vi "to string.vi"(8 "error in":errorcluster, 11 "Thermo Channel configuration":refnum<class "Thermo Channel configuration.lvclass">) -> (0 "error out":errorcluster, 1 "data":string, 2 "version":string, 3 "Thermo Channel configuration out":refnum<class "Thermo Channel configuration.lvclass">)   [LabVIEW 2025, in "Thermo.lvlib" / "Thermo Channel configuration.lvclass"]
doc: "Provides an interface for saving a module configuration to a file or other serialized data source. It is recommended that all children of this class store data in two sets--data required for its own initialization, and any data required for parent initialization--and that each implementation uses the <b>Call Parent Method</b> primitive to serialize parent information.Copyright 2017 National Instruments Corporation\n\nLicensed under the Apache License, Version 2.0 (the \"License\"); you may not use this file except in compliance with the License. You may obtain a copy of the License at http://www.apache.org/licenses/LICENSE-2.0\nUnless required by applicable law or agreed to in writing, software distributed under the License is distributed on an \"AS IS\" BASIS, WITHOUT WARRANTIES OR CONDITIONS OF ANY KIND, either express or implied. See the License for the specific language governing permissions and limitations under the License."
uses:
  Thermo Channel configuration.lvclass
  C:/Users/Public/Documents/Sandia National Labs/TSS Plugin/Abstract Engine.lvlibp/Plugin/Abstract/Channel configuration/Channel configuration.lvclass
  Thermo Channel configuration.lvclass/Thermo Channel configuration.ctl
  Read Thermo Channel.vi
  Users/Public/Documents/Sandia National Labs/TSS Plugin/Abstract Engine.lvlibp/Plugin/Abstract/Channel configuration/Read Channel Setting.vi
  Users/Public/Documents/Sandia National Labs/TSS Plugin/Abstract Engine.lvlibp/Plugin/Abstract/Channel configuration/Channel configuration.lvclass
  Users/Public/Documents/Sandia National Labs/TSS Plugin/CEF.lvlibp/serializable configuration/CEF_serializable configuration.lvclass
  Users/Public/Documents/Sandia National Labs/TSS Plugin/CEF.lvlibp
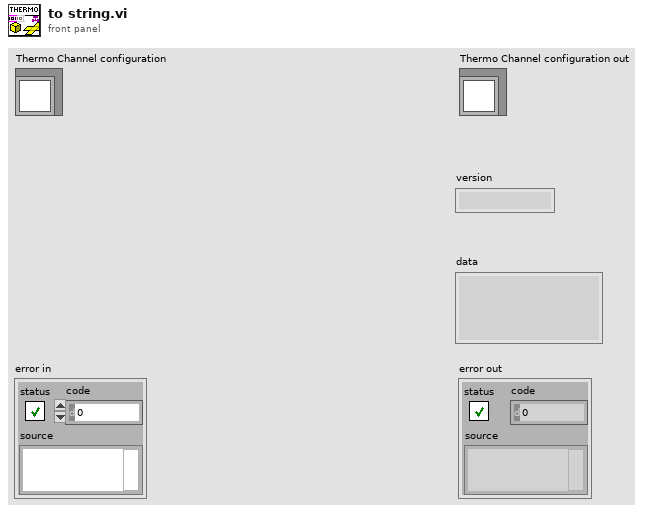
[diagram p1: front panel]
types:
  T1 = typedef "Thermo.lvlib/Thermo Channel configuration.lvclass/Channel Setting.ctl" = cluster{"Numeric":dbl, "Combo":string, "String":string, "Boolean":bool}
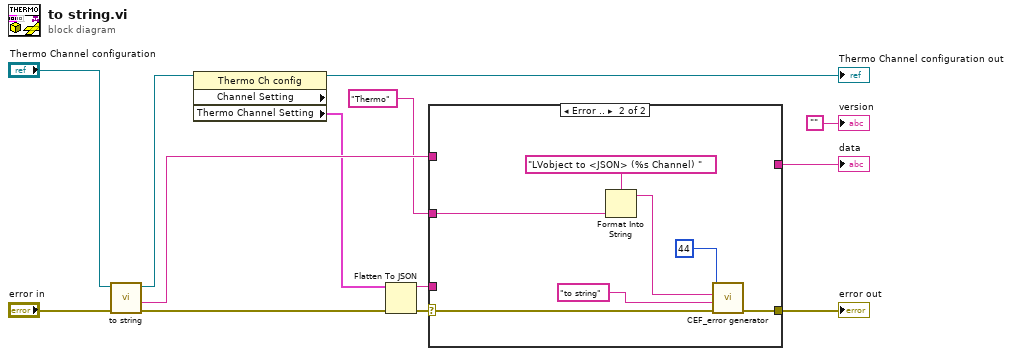
[diagram p0: block diagram]
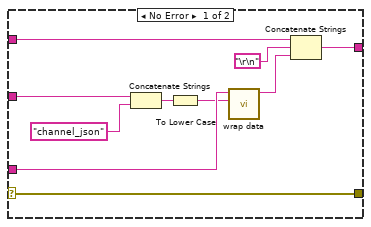
[diagram p2: hidden frame]
diagram:
  n1 = call-parent "to string.vi"("error in"="error in", "Channel configuration"="Thermo Channel configuration") -> ("error out"=w8:errorcluster, "data"=w4:string, "Channel configuration out"=w6:refnum<class "Thermo Channel configuration.lvclass">)  [unwired: 6 in, 1 out]
  n2 = property class="Thermo Ch config" props=["Channel Setting", "Thermo Channel Setting"](reference=w6) -> (reference out=→"Thermo Channel configuration out":refnum<class "Thermo Channel configuration.lvclass">, "Thermo Channel Setting"=w2:T1)  [unwired: 1 in, 2 out]
  n3 = Flatten To JSON(anything=w2, error in (no error)=w8) -> (JSON string=w10:string, 11:w9:errorcluster)  [unwired: 1 in]
  n4 = case shown="Error .." w9 {
    selector: w9 -> [w23 w28]
    tunnel: [w23 w27] -> w7
    tunnel: w10 -> [w21 _]
    tunnel: w4 -> [w20 _]
    tunnel: [w18 _] -> w5
    tunnel: "Thermo" ("additional identifier") -> [w16 w24]
    frame No Error {
      n5 = Concatenate Strings(w16, "channel_json" ("additional identifier")) -> (w14:string)
      n6 = To Lower Case(string=w14) -> (all lower case string=w17:string)
      n7 = call "wrap data.vi"("identifier"=w17, "data to wrap"=w21) -> ("wrapped data"=w22:string)  [unwired: 9 in]
      n8 = Concatenate Strings(w20, "\r\n", w22) -> (w18:string)
    }
    frame Error {
      n9 = Format Into String(format string="LVobject to <JSON> (%s Channel) " ("message"), w24) -> (resulting string=w25:string)  [unwired: 2 in, 1 out]
      n10 = call "CEF_error generator.vi"("error in"=w28, "source"="to string" ("message"), "append error message"=w25, "error code (0)"=44) -> ("error out"=w27:errorcluster)  [unwired: 5 in]
    }
  }
  "error out" <- w7
  "data" <- w5
  "version" <- ""
